vi "Convert to Array Data in Single Current Mode_BU.vi"() -> ()   [LabVIEW 2023]
panel:
  in  "External\nRef":bool=TRUE
  in  "x/y":dbl[](array[numeric])
  in  "subarray":u8[](array[numeric])
  in  "Electrode number, N":u16=8
  in  "Array Mode":u16(ring) items=["Gradient + Dipole dipole", "Gradient", "Dipole Dipole", "Schlumberger"]
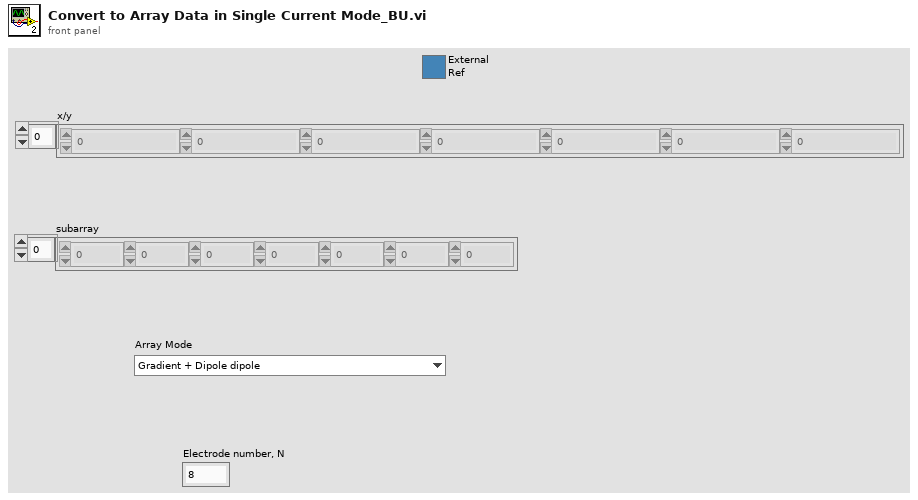
[diagram p1: front panel]
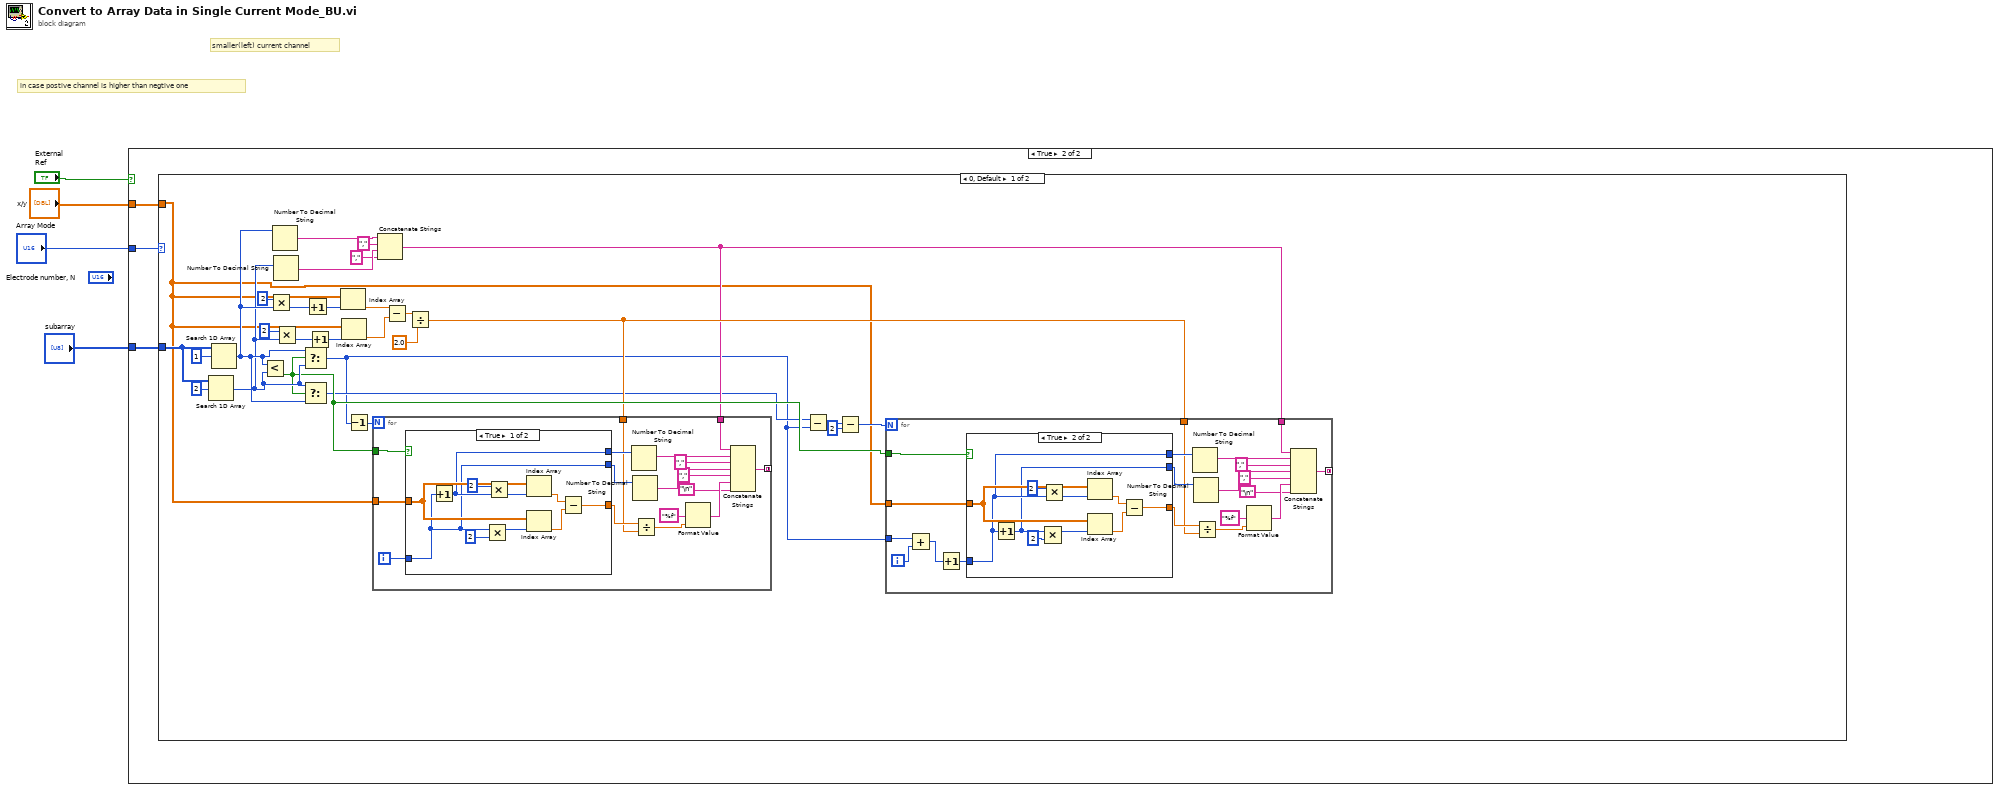
[diagram p0: block diagram]
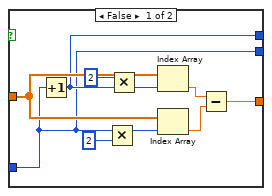
[diagram p3: hidden frame]
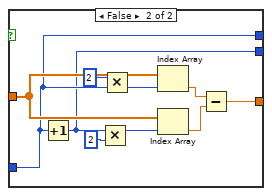
[diagram p4: hidden frame]
diagram:
  # "smaller(left) current channel"
  # "in case postive channel is higher than negtive one"
  n1 = case shown="True" "External\nRef" {
    tunnel: "Array Mode" -> [_ w7]
    tunnel: "subarray" -> [_ w6]
    tunnel: "x/y" -> [_ w5]
    frame False {
    }
    frame True {
      n2 = case shown="0, Default" w7 {
        tunnel: w6 -> [w34 _]
        tunnel: w5 -> [w10 _]
        frame 0, Default {
          n3 = Search 1D Array(1D array=w34, element=u8 2) -> (index of element=w27:i32)  [unwired: 1 in]
          n4 = Search 1D Array(1D array=w34, element=u8 1) -> (index of element=w28:i32)  [unwired: 1 in]
          n5 = Less?(x=w28, y=w27) -> (x < y?=w13:bool)
          n6 = Multiply(x=2, y=w28) -> (x*y=w22:i32)
          n7 = Number To Decimal String(number=w28) -> (decimal integer string=w32:string)  [unwired: 1 in]
          n8 = Number To Decimal String(number=w27) -> (decimal integer string=w30:string)  [unwired: 1 in]
          n9 = Multiply(x=2, y=w27) -> (x*y=w19:i32)
          n10 = Select(t=w28, s=w13, f=w27) -> (s? t:f=w8:i32)
          n11 = Select(t=w27, s=w13, f=w28) -> (s? t:f=w9:i32)
          n12 = Increment(x=w22) -> (x+1=w20:i32)
          n13 = Increment(x=w19) -> (x+1=w17:i32)
          n14 = Index Array(array=w10, index=w20) -> (element=w26:dbl)
          n15 = Index Array(array=w10, index=w17) -> (element=w25:dbl)
          n16 = Decrement(x=w8) -> (x-1=w33:i32)
          n17 = Concatenate Strings(w32, "," ("string"), w30, "," ("string")) -> (w11:string)
          n18 = Subtract(x=w26, y=w25) -> (x-y=w24:dbl)
          n19 = Divide(x=w24, y=2.0) -> (x/y=w12:dbl)
          n20 = for {
            N: w33 -> [_]
            tunnel: w13 -> [w93]
            tunnel: w10 -> [w92]
            tunnel: w11 -> [w83]
            tunnel: w12 -> [w81]
            tunnel: [w77] -> _ mode=concatenating
            i -> [w91]
            n21 = case shown="True" w93 {
              tunnel: w92 -> [w103 w113]
              tunnel: w91 -> [w98 w109]
              tunnel: [w100 w110] -> w82
              tunnel: [w99 w109] -> w90
              tunnel: [w98 w108] -> w89
              frame True {
                n22 = Increment(x=w98) -> (x+1=w99:i32)
                n23 = Multiply(x=w98, y=2) -> (x*y=w95:i32)
                n24 = Multiply(x=2, y=w99) -> (x*y=w97:i32)
                n25 = Index Array(array=w103, index=w97) -> (element=w102:dbl)
                n26 = Index Array(array=w103, index=w95) -> (element=w101:dbl)
                n27 = Subtract(x=w102, y=w101) -> (x-y=w100:dbl)
              }
              frame False {
                n28 = Increment(x=w109) -> (x+1=w108:i32)
                n29 = Multiply(x=w108, y=2) -> (x*y=w105:i32)
                n30 = Multiply(x=2, y=w109) -> (x*y=w107:i32)
                n31 = Index Array(array=w113, index=w107) -> (element=w112:dbl)
                n32 = Index Array(array=w113, index=w105) -> (element=w111:dbl)
                n33 = Subtract(x=w112, y=w111) -> (x-y=w110:dbl)
              }
            }
            n34 = Number To Decimal String(number=w90) -> (decimal integer string=w87:string)  [unwired: 1 in]
            n35 = Number To Decimal String(number=w89) -> (decimal integer string=w85:string)  [unwired: 1 in]
            n36 = Divide(x=w82, y=w81) -> (x/y=w80:dbl)
            n37 = Format Value(format string="%f", value (0)=w80) -> (output string=w79:string)  [unwired: 1 in]
            n38 = Concatenate Strings(w83, w87, "," ("string"), w85, "," ("string"), w79, "\n") -> (w77:string)
          }
          n39 = Subtract(x=w9, y=w8) -> (x-y=w16:i32)
          n40 = Subtract(x=w16, y=2) -> (x-y=w14:i32)
          n41 = for {
            N: w14 -> [_]
            tunnel: w13 -> [w56]
            tunnel: w10 -> [w55]
            tunnel: w11 -> [w47]
            tunnel: w12 -> [w45]
            tunnel: [w41] -> _ mode=concatenating
            tunnel: w8 -> [w40]
            i -> [w39]
            n42 = Add(x=w40, y=w39) -> (x+y=w38:i32)
            n43 = Increment(x=w38) -> (x+1=w37:i32)
            n44 = case shown="True" w56 {
              tunnel: w55 -> [w66 w76]
              tunnel: w37 -> [w61 w72]
              tunnel: [w63 w73] -> w46
              tunnel: [w62 w72] -> w54
              tunnel: [w61 w71] -> w53
              frame False {
                n45 = Increment(x=w61) -> (x+1=w62:i32)
                n46 = Multiply(x=w61, y=2) -> (x*y=w58:i32)
                n47 = Multiply(x=2, y=w62) -> (x*y=w60:i32)
                n48 = Index Array(array=w66, index=w60) -> (element=w65:dbl)
                n49 = Index Array(array=w66, index=w58) -> (element=w64:dbl)
                n50 = Subtract(x=w65, y=w64) -> (x-y=w63:dbl)
              }
              frame True {
                n51 = Increment(x=w72) -> (x+1=w71:i32)
                n52 = Multiply(x=w71, y=2) -> (x*y=w68:i32)
                n53 = Multiply(x=2, y=w72) -> (x*y=w70:i32)
                n54 = Index Array(array=w76, index=w70) -> (element=w75:dbl)
                n55 = Index Array(array=w76, index=w68) -> (element=w74:dbl)
                n56 = Subtract(x=w75, y=w74) -> (x-y=w73:dbl)
              }
            }
            n57 = Number To Decimal String(number=w54) -> (decimal integer string=w51:string)  [unwired: 1 in]
            n58 = Number To Decimal String(number=w53) -> (decimal integer string=w49:string)  [unwired: 1 in]
            n59 = Divide(x=w46, y=w45) -> (x/y=w44:dbl)
            n60 = Format Value(format string="%f", value (0)=w44) -> (output string=w43:string)  [unwired: 1 in]
            n61 = Concatenate Strings(w47, w51, "," ("string"), w49, "," ("string"), w43, "\n") -> (w41:string)
          }
        }
        frame 1 {
        }
      }
    }
  }
